vi "wsCallService.vi"(8 "error in (no error)":errorcluster, 10 "Call Service Data":T1, 11 "References":T2) -> (0 "error out":errorcluster, 3 "Success?":bool)   [LabVIEW 2018, in "HASS-LV-WS_integration.lvlib"]
uses:
  HASS-LV-WS_integration.lvlib
  TypeDef/ReferencesTypeDef.ctl
  TypeDef/QueueTypeDef.ctl
  TypeDef/EventTypeDef.ctl
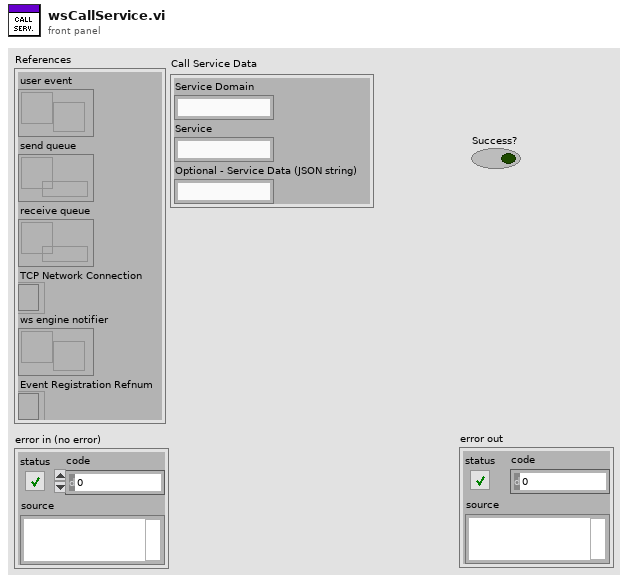
[diagram p1: front panel]
types:
  T1 = cluster{"Service Domain":string, "Service":string, "Optional - Service Data (JSON string)":string}
  T2 = typedef "HASS-LV-WS_integration.lvlib/ReferencesTypeDef.ctl" = cluster{"user event":refnum<user-event>, "send queue":refnum<queue>, "receive queue":refnum<queue>, "TCP Network Connection":refnum<k5>, "ws engine notifier ":refnum<notifier>, "Event Registration Refnum":refnum<event-registration>}
  T3 = typedef "HASS-LV-WS_integration.lvlib/EventTypeDef.ctl" = cluster{"Data":variant, "Command":string}
  T4 = cluster{"id":i32, "type":string, "domain":string, "service":string}
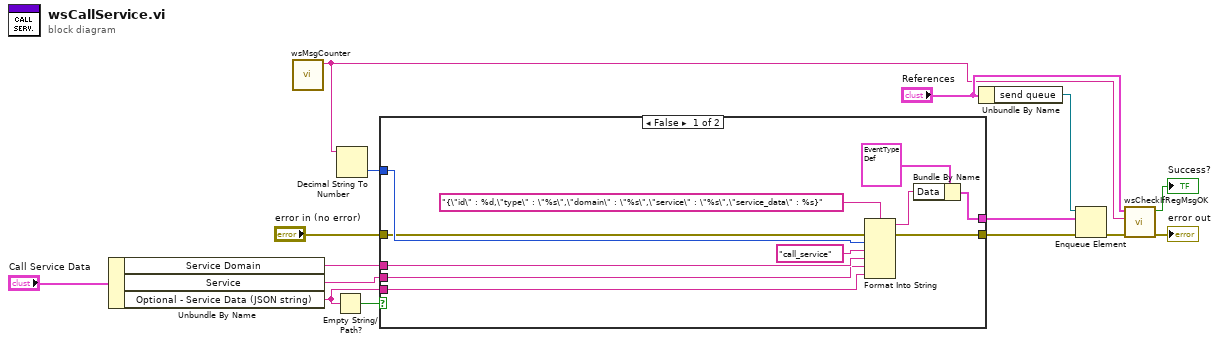
[diagram p0: block diagram]
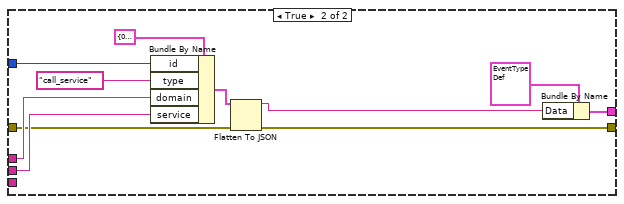
[diagram p2: hidden frame]
diagram:
  n1 = Unbundle By Name("Call Service Data") -> ("Service Domain"=w5:string, "Service"=w4:string, "Optional - Service Data (JSON string)"=w3:string)
  n2 = call "wsMsgCounter.vi"() -> ("msgCounter"=w13:string)  [unwired: 11 in]
  n3 = Empty String/Path?(string/path=w3) -> (empty?=w11:bool)
  n4 = Decimal String To Number(string=w13) -> (number=w12:i32)  [unwired: 2 in, 1 out]
  n5 = case shown="False" w11 {
    tunnel: w12 -> [w23 w36]
    tunnel: w5 -> [w21 w35]
    tunnel: w4 -> [w20 w34]
    tunnel: w3 -> [w19 _]
    tunnel: [w25 w31] -> w10
    tunnel: "error in (no error)" -> [w18 w27]
    tunnel: [w17 w28] -> w1
    frame False {
      n6 = Format Into String(format string="{\"id\" : %d,\"type\" : \"%s\",\"domain\" : \"%s\",\"service\" : \"%s\",\"service_data\" : %s}", error in=w18, w23, "call_service" ("type"), w21, w20, w19) -> (resulting string=w16:string, error out=w17:errorcluster)  [unwired: 1 in]
      n7 = Bundle By Name(cluster=T3 {"Data"=variant, "Command"="Send"} ("element"), "Data"=w16) -> (w25:T3)
    }
    frame True {
      n8 = Bundle By Name(cluster=T4 {"id"=0, "type"="", "domain"="", "service"=""}, "id"=w36, "type"="call_service", "domain"=w35, "service"=w34) -> (w30:T4)
      n9 = Flatten To JSON(anything=w30, error in (no error)=w27) -> (JSON string=w29:string, 11:w28:errorcluster)  [unwired: 1 in]
      n10 = Bundle By Name(cluster=T3 {"Data"=variant, "Command"="Send"} ("element"), "Data"=w29) -> (w31:T3)
    }
  }
  n11 = Unbundle By Name("References") -> ("send queue"=w15:refnum<queue>)
  n12 = Enqueue Element(queue=w15, element=w10, error in (no error)=w1) -> (error out=w9:errorcluster)  [unwired: 1 in, 2 out]
  n13 = call "wsCheckIfRegMsgOK.vi"("error in (no error)"=w9, "msgCounter"=w13, "References"="References") -> ("error out"=→"error out":errorcluster, "Success?"=→"Success?":bool)  [unwired: 6 in, 1 out]
